vi "WriteArea.vi"() -> ()   [LabVIEW 2014]
uses:
  lib/Snap7.lvlib
panel:
  out "Result":i32
  in  "data in":string
  out "?":string
  out "Running":bool
  out "Status":string="No Error"
  in  "Word Length":i32(ring)=2 items=["Bit"=1, "Byte"=2, "Word"=4, "DWord"=6, "Real"=8, "Counter"=28, "Timer"=29]
  in  "Area":i32(ring)=132 items=["Inputs (EB)"=129, "Output (AB)"=130, "Bit Memory (M)"=131, "Data (DB)"=132, "Counters (Z)"=28, "Timers (T)"=29]
  in  "Amount":i32=16
  in  "Start":i32
  in  "DB Number":i32=1
  in  "?":bool
  in  "Slot":i32=2
  in  "Rack":i32
  in  "Address IP":string="192.168.1.12"
  # "Data Read"
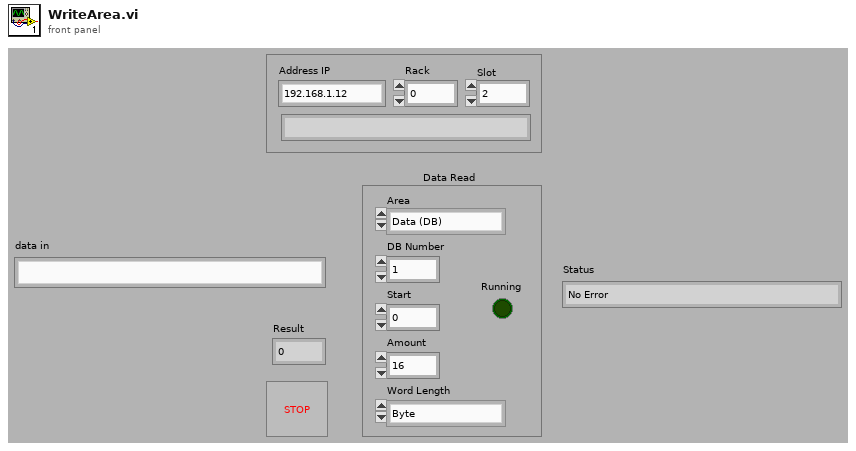
[diagram p1: front panel]
types:
  T1 = enum16{"big-endian, network order", "native, host order", "little-endian"}
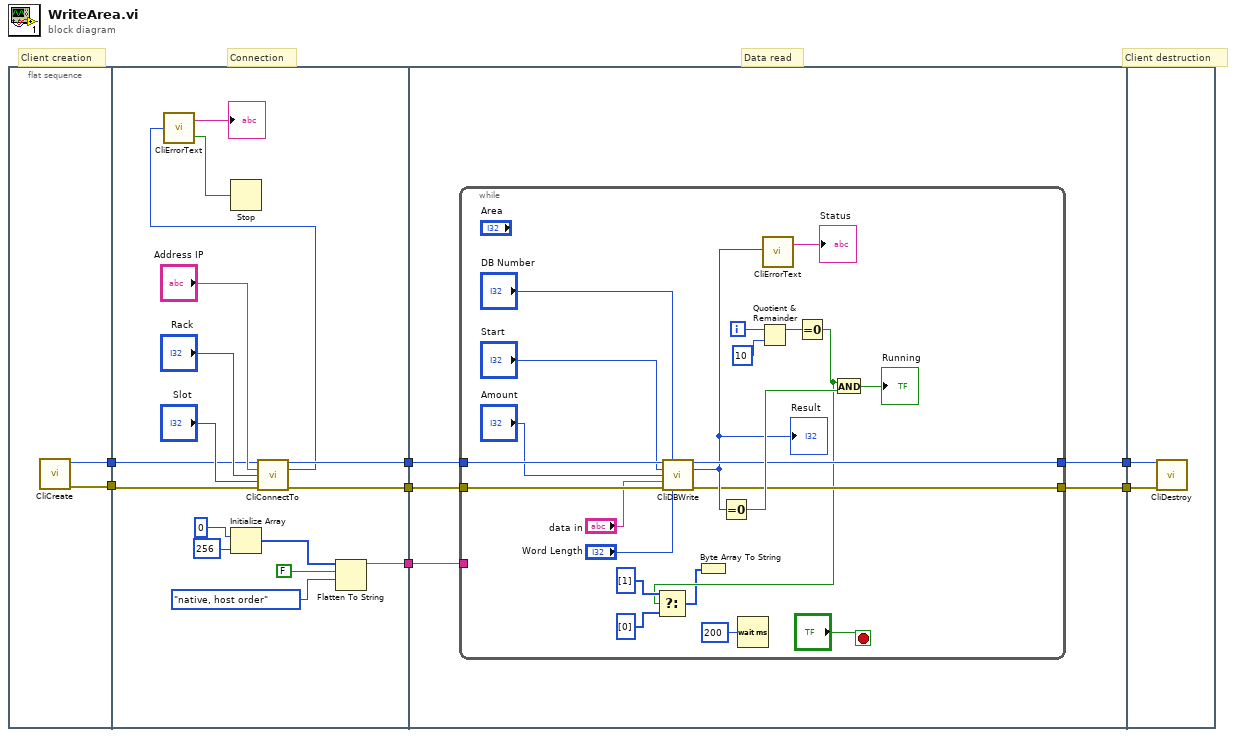
[diagram p0: block diagram]
diagram:
  # "Client destruction"
  # "Data read"
  # "Connection"
  # "Client creation"
  n1 = flat-sequence {
    tunnel: [w9] -> w4
    tunnel: [w8] -> w3
    tunnel: [w20] -> w7
    tunnel: [w13] -> w6
    tunnel: [w19] -> w5
    tunnel: w4 -> [w15]
    tunnel: w3 -> [w14]
    tunnel: w7 -> [w30]
    tunnel: w6 -> [w29]
    tunnel: w5 -> [w28]
    tunnel: [w27] -> w2
    tunnel: [w26] -> w1
    tunnel: w2 -> [w54]
    tunnel: w1 -> [w53]
    frame #0 {
      n2 = call "CliCreate.vi"() -> ("ref out"=w9:u64, "error out"=w8:errorcluster)  [unwired: 14 in]
    }
    frame #1 {
      n3 = Initialize Array(u8 0, 256) -> (w23:u8[])
      n4 = call "CliConnectTo.vi"("ref in"=w15, "Address"="Address IP", "Rack"="Rack", "Slot"="Slot", "error in (no error)"=w14) -> ("ref out"=w13:u64, "Result"=w10:i32, "error out"=w20:errorcluster)  [unwired: 8 in]
      n5 = call "CliErrorText.vi"("ErrNo"=w10) -> ("Error"=w11:bool, "ErrMessage"=→"?":string)
      n6 = Stop(stop? (T)=w11) -> ()
      n7 = Flatten To String(anything=w23, prepend array or string size? (T)=FALSE, byte order (0:big-endian, network order)=T1."native, host order") -> (data string=w19:string)  [unwired: 1 in, 2 out]
    }
    frame #2 {
      n8 = while {
        tunnel: w30 -> [w38]
        tunnel: w29 -> [w44]
        tunnel: w28 -> [_]
        tunnel: [w40] -> w27
        tunnel: [w37] -> w26
        i -> [w51]
        stop <- "?" stop-if-true
        n9 = call "CliDBWrite.vi"("ref in"=w44, "DB Number"="DB Number", "Start"="Start", "Amount"="Amount", "data in"="data in", "error in (no error)"=w38, "Word Length"="Word Length") -> ("ref out"=w40:u64, "Result"=w39:i32, "error out"=w37:errorcluster)  [unwired: 6 in]
        "Result" <- w39
        n10 = Equal To 0?(x=w39) -> (x = 0?=w47:bool)
        n11 = Wait (ms)(milliseconds to wait=u32 200) -> ()  [unwired: 1 out]
        n12 = Quotient & Remainder(x=w51, y=10) -> (x-y*floor(x/y)=w49:i32)  [unwired: 1 out]
        n13 = call "CliErrorText.vi"("ErrNo"=w39) -> ("ErrMessage"=→"Status":string)  [unwired: 1 out]
        n14 = Equal To 0?(x=w49) -> (x = 0?=w34:bool)
        n15 = Select(t=u8[] [1] ("ByteData"), s=w34, f=u8[] [0] ("ByteData")) -> (s? t:f=w33:u8[])
        n16 = Byte Array To String(unsigned byte array=w33) -> ()  [unwired: 1 out]
        n17 = And(x=w34, y=w47) -> (x .and. y?=→"Running":bool)
      }
    }
    frame #3 {
      n18 = call "CliDestroy.vi"("ref in"=w54, "error in (no error)"=w53) -> ()  [unwired: 13 in, 1 out]
    }
  }
